vi "dfd_FXP Sub (vv).vi"(4 "quantization settings":T4={"source"=6, "wl"=1, "iwl"=1, "overflow mode"=enum."Saturation", "rounding mode"=enum."Nearest", "signed?"=TRUE} {"source" items=["Coefficients a/k"=0, "Coefficients b/v"=7, "Input"=1, "Output"=2, "Multiplicand"=3, "Product"=4, "Sum"=5, "Delay"=6]}, 5 "filtering statistics in":T3(array[cluster]) {"statistics information"."min value" format="%.2f"; "statistics information"."max value" format="%.2f"; "Quantizer Source" items=["Coefficients a/k"=0, "Coefficients b/v"=7, "Input"=1, "Output"=2, "Multiplicand"=3, "Product"=4, "Sum"=5, "Delay"=6]}, 7 "values2 in":dbl[](array[numeric]) format="%.2f", 8 "values1 in":dbl[](array[numeric]) format="%.2f") -> (0 "filtering statistics out":T3(array[cluster]) {"statistics information"."min value" format="%.2f"; "statistics information"."max value" format="%.2f"; "Quantizer Source" items=["Coefficients a/k"=0, "Coefficients b/v"=7, "Input"=1, "Output"=2, "Multiplicand"=3, "Product"=4, "Sum"=5, "Delay"=6]}, 2 "statistics information":T2 {"min value" format="%.2f"; "max value" format="%.2f"}, 3 "values out":dbl[](array[numeric]) format="%.2f")   [LabVIEW 2017, in "NI_DigFilter_FXP.lvlib"]
uses:
  <vilib>/addons/Digital Filter Design/NI_DigFilter_FXP.lvlib
  <vilib>/addons/Digital Filter Design/_Objects.llb/DFD Quantization Settings.ctl
  <vilib>/addons/Digital Filter Design/_Objects.llb/DFD Quantization Sources.ctl
  <vilib>/addons/Digital Filter Design/_Objects.llb/DFD FXP Statistics Data.ctl
  <vilib>/addons/Digital Filter Design/FXPLib.llb/dfd_FXP Casting (vector).vi
  <vilib>/addons/Digital Filter Design/NI_DigFilterLicensed.lvlib
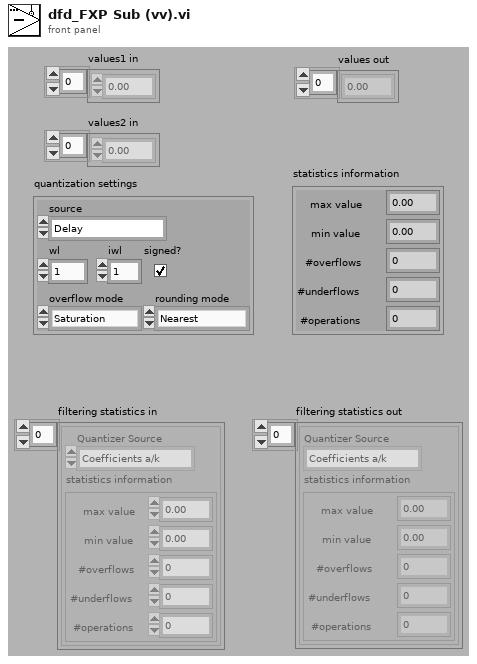
[diagram p1: front panel]
types:
  T1 = typedef "NI_DigFilterLicensed.lvlib/DFD Quantization Sources.ctl" = u16
  T2 = typedef "NI_DigFilterLicensed.lvlib/DFD FXP Statistics Data.ctl" = cluster{"max value":ext, "min value":ext, "#overflows":i32, "#underflows":i32, "#operations":i32}
  T3 = cluster{"Quantizer Source":T1, "statistics information":T2}[]
  T4 = typedef "NI_DigFilterLicensed.lvlib/DFD Quantization Settings.ctl" = cluster{"source":T1, "wl":i16, "iwl":i16, "overflow mode":enum16{"Saturation", "Wrap"}, "rounding mode":enum16{"Nearest", "Truncation"}, "signed?":bool}
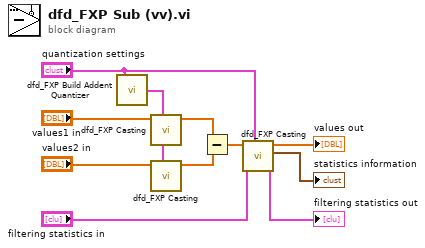
[diagram p0: block diagram]
diagram:
  n1 = call <vilib>:"dfd_FXP Build Addent Quantizer.vi"("sum quantizer"="quantization settings") -> ("addent quantizer"=w3:T4)
  n2 = call-poly <vilib>:"dfd_FXP Casting.vi"("quantization settings"=w3, "values in"="values1 in") -> ("values out"=w7:dbl[])  [unwired: 1 in, 6 out]
  n3 = call-poly <vilib>:"dfd_FXP Casting.vi"("quantization settings"=w3, "values in"="values2 in") -> ("values out"=w5:dbl[])  [unwired: 1 in, 6 out]
  n4 = Subtract(x=w7, y=w5) -> (x-y=w11:dbl[])
  n5 = call-poly <vilib>:"dfd_FXP Casting.vi"("quantization settings"="quantization settings", "filtering statistics in"="filtering statistics in", "values in"=w11) -> ("filtering statistics out"=→"filtering statistics out":T3, "statistics information"=→"statistics information":T2, "values out"=→"values out":dbl[])  [unwired: 4 out]
